vi "SlowAO_duration.vi"(1 "Slow AO Array":T1 {"Duration, Gain, NewVal" format="%#_3g"}) -> (0 "Duration (s)":dbl=0.1)   [LabVIEW 2018]
uses:
  ParameterSubCluster.ctl
panel:
  in  "lower limit":dbl=0.1
  in  "upper limit":dbl=1000000.0
  # "don't go lower than 0.1 s or something\n(otherwise might divide by 0 if empty array)\n\nthe sky is the upper limit. I can just see\nsomebody asking me to do a 1 hour wait"
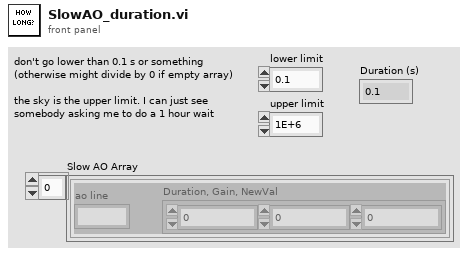
[diagram p1: front panel]
types:
  T1 = typedef "ParameterSubCluster.ctl" = cluster{"ao line":string, "Duration, Gain, NewVal":dbl[]}[]
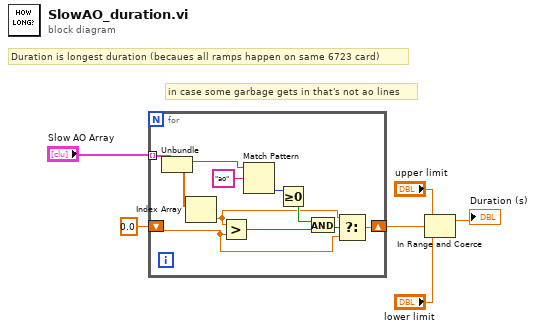
[diagram p0: block diagram]
diagram:
  # "Duration is longest duration (becaues all ramps happen on same 6723 card)"
  # "in case some garbage gets in that's not ao lines"
  n1 = for {
    tunnel: "Slow AO Array" -> [w17] mode=indexing
    shift-right: [w9] -> w5
    shift-left: 0.0 -> [w7]
    n2 = Unbundle(w17) -> ("ao line"=w15:string, "Duration, Gain, NewVal"=w16:dbl[])
    n3 = Index Array(array=w16) -> (element=w8:dbl)  [unwired: 1 in]
    n4 = Greater?(x=w8, y=w7) -> (0:w11:bool)
    n5 = Match Pattern(string=w15, regular expression="ao") -> (offset past match=w13:i32)  [unwired: 1 in, 3 out]
    n6 = Greater Or Equal To 0?(x=w13) -> (x >= 0?=w12:bool)
    n7 = And(x=w12, y=w11) -> (x .and. y?=w10:bool)
    n8 = Select(t=w8, s=w10, f=w7) -> (s? t:f=w9:dbl)
  }
  n9 = In Range and Coerce(upper limit="upper limit", x=w5, lower limit="lower limit") -> (coerced(x)=→"Duration (s)":dbl)  [unwired: 1 out]
